vi "Constants.vi"() -> ()   [LabVIEW 2016, in "FPGA Resource Manager Client Example Shared.lvlib"]
doc: "Use this Global VI to access the GUIDs assigned to the page resources of the Custom Device."
uses:
  FPGA Resource Manager Client Example Shared.lvlib
panel:
  in  "Tab Control":enum32{"GUIDS", "Constants", "Properties"}(tab)
  in  "FPGA Resource Manager Client Example":string="0325c7a6-2035-4d79-9062-56d59de9d05c"
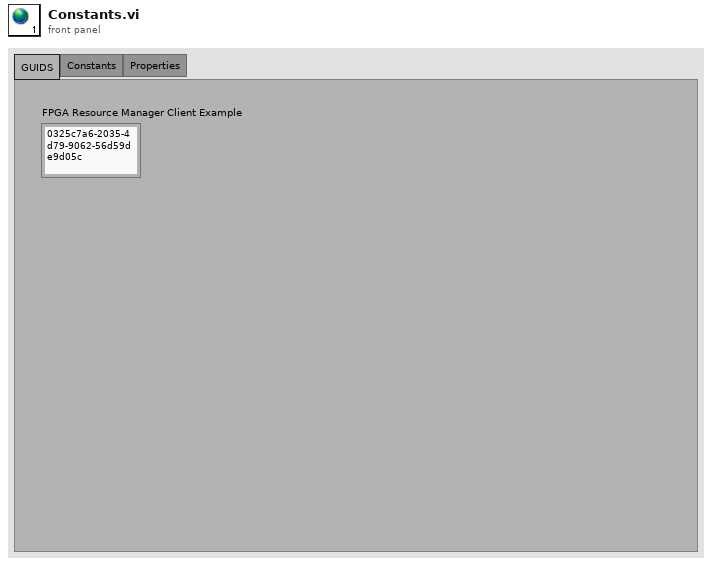
[diagram p1: front panel]
diagram:
